vi "Set Speed.vi"(8 "error in (no error)":errorcluster, 10 "speed":dbl, 11 "EPOS4 Settings In":T2={"VISA resource name"="", "axis"={"keyHandle"=0, "nodeId"=1}, "Simulated?"=FALSE}) -> (0 "error out":errorcluster, 1 "Connection Error":bool, 3 "EPOS4 Settings Out":T2={"VISA resource name"="", "axis"={"keyHandle"=0, "nodeId"=1}, "Simulated?"=FALSE})   [LabVIEW 2018, in "EPOS4.lvlib"]
uses:
  EPOS4.lvlib
  Controls/EPOS Communication Settings.ctl
panel:
  in  "timeout":u32=1000
  in  "velocity profile":T1={"profileAcceleration"=10000, "profileDeceleration"=10000}
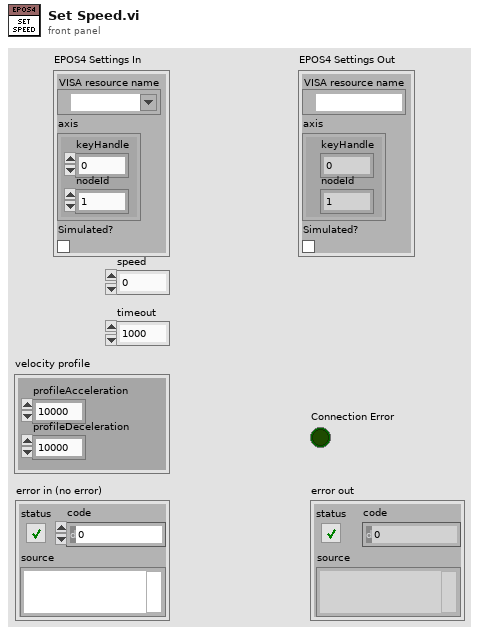
[diagram p1: front panel]
types:
  T1 = cluster{"profileAcceleration":u32, "profileDeceleration":u32}
  T2 = typedef "EPOS4.lvlib/EPOS Communication Settings.ctl" = cluster{"VISA resource name":refnum<visa-resource-name>, "axis":cluster{"keyHandle":u32, "nodeId":u16}, "Simulated?":bool}
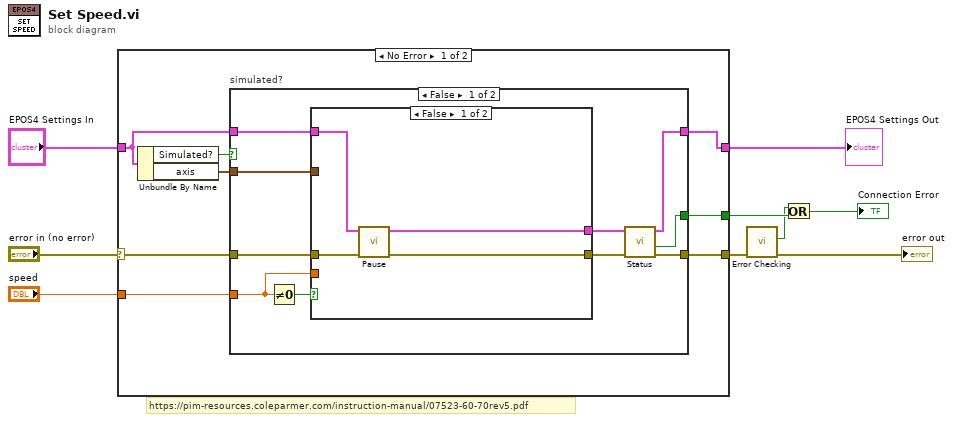
[diagram p0: block diagram]
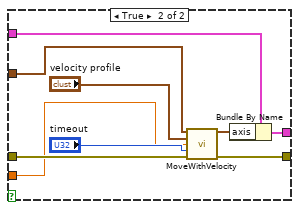
[diagram p2: hidden frame]
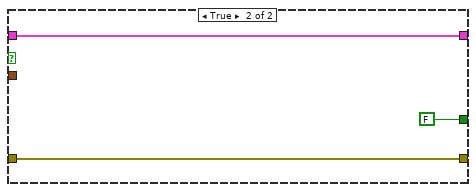
[diagram p3: hidden frame]
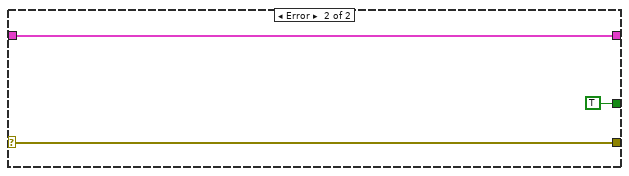
[diagram p4: hidden frame]
diagram:
  # "https://pim-resources.coleparmer.com/instruction-manual/07523-60-70rev5.pdf"
  n1 = case shown="No Error" "error in (no error)" {
    selector: "error in (no error)" -> [w17 w46]
    tunnel: [w16 w46] -> w9
    tunnel: [w10 w45] -> w1
    tunnel: "EPOS4 Settings In" -> [w13 w45]
    tunnel: "speed" -> [w15 _]
    tunnel: [w14 TRUE ("Connection Error")] -> w5
    frame No Error {
      n2 = Unbundle By Name(w13) -> ("Simulated?"=w12:bool, "axis"=w11:cluster{"keyHandle":u32, "nodeId":u16})
      n3 = case "simulated?" shown="False" w12 {
        tunnel: w17 -> [w26 w43]
        tunnel: [w21 w43] -> w16
        tunnel: w11 -> [w27 _]
        tunnel: w15 -> [w19 _]
        tunnel: w13 -> [w25 w41]
        tunnel: [w20 FALSE ("Connection Error")] -> w14
        tunnel: [w22 w41] -> w10
        frame False {
          n4 = Not Equal To 0?(x=w19) -> (x != 0?=w18:bool)
          n5 = case shown="False" w18 {
            tunnel: w27 -> [_ w38]
            tunnel: w26 -> [w29 w37]
            tunnel: w25 -> [w30 w36]
            tunnel: [w28 w34] -> w24
            tunnel: [w31 w33] -> w23
            tunnel: w19 -> [_ w32]
            frame False {
              n6 = call "Pause.vi"("error in (no error)"=w29, "EPOS4 Settings in"=w30) -> ("error out"=w28:errorcluster, "EPOS4 Settings out"=w31:T2)  [unwired: 7 in, 1 out]
            }
            frame True {
              n7 = call "MoveWithVelocity.vi"("axis in"=w38, "velocity profile"="velocity profile", "targetVelocity"=w32, "timeout"="timeout", "error in (no error)"=w37) -> ("axis out"=w35:cluster{"keyHandle":u32, "nodeId":u16}, "error out"=w34:errorcluster)  [unwired: 9 in]
              n8 = Bundle By Name(cluster=w36, "axis"=w35) -> (w33:T2)
            }
          }
          n9 = call "Status.vi"("error in (no error)"=w24, "EPOS4 Settings In"=w23) -> ("error out"=w21:errorcluster, "Connection Error"=w20:bool, "EPOS4 Settings Out"=w22:T2)  [unwired: 5 in, 2 out]
        }
        frame True {
        }
      }
    }
    frame Error {
    }
  }
  "EPOS4 Settings Out" <- w1
  n10 = call "Error Checking.vi"("error in (no error)"=w9) -> ("error out"=→"error out":errorcluster, "Connection Error"=w2:bool)  [unwired: 8 in, 1 out]
  n11 = Or(x=w2, y=w5) -> (x .or. y?=→"Connection Error":bool)
